vi "Add Station Information.vi"(8 "error in (no error)":errorcluster, 10 "Station Info":T1, 11 "OnTheFlyReport in":refnum<class "OnTheFlyReport.lvclass">) -> (0 "error out":errorcluster, 3 "OnTheFlyReport out":refnum<class "OnTheFlyReport.lvclass">)   [LabVIEW 2015, in "OnTheFlyReport.lvclass"]
doc: "This VI takes Station Information and saves it to the permanent report"
uses:
  OnTheFlyReport.lvclass
  Report Information/Station Information.ctl
  OnTheFlyReport.lvclass/OnTheFlyReport.ctl
  Report Formatters/Base Class/Execution/Formatter.lvclass
  Report Information/Report Information.lvclass
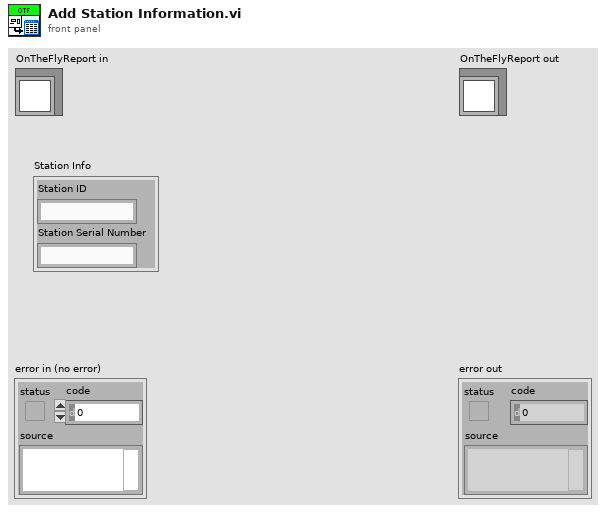
[diagram p1: front panel]
types:
  T1 = typedef "Report Information.lvclass/Station Information.ctl" = cluster{"Station ID":string, "Station Serial Number":string}
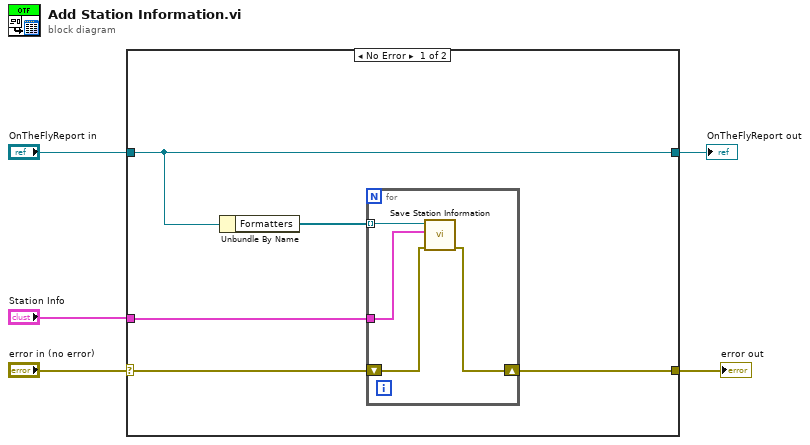
[diagram p0: block diagram]
diagram:
  n1 = case shown="No Error" "error in (no error)" {
    selector: "error in (no error)" -> [w8 w16]
    tunnel: [w7 w16] -> w4
    tunnel: [w6 w15] -> w3
    tunnel: "OnTheFlyReport in" -> [w6 w15]
    tunnel: "Station Info" -> [w9 _]
    frame No Error {
      n2 = Unbundle By Name(w6) -> ("Formatters"=w10:refnum<class "Formatter.lvclass">[])
      n3 = for {
        tunnel: w10 -> [w14] mode=indexing
        tunnel: w9 -> [w13]
        shift-right: [w11] -> w7
        shift-left: w8 -> [w12]
        n4 = call-dynamic "Save Station Information.vi"("error in (no error)"=w12, "Station Info"=w13, "Formatter in"=w14) -> ("error out"=w11:errorcluster)  [unwired: 7 in, 1 out]
      }
    }
    frame Error {
    }
  }
  "error out" <- w4
  "OnTheFlyReport out" <- w3
